vi "Append Paragraph.vi"(0 "PDF Report":T24(xcontrol), 2 "Text":string, 3 "Paragraph indentation":T3, 7 "Image to Add [ ]":T1 {"Scale" format="%#_g %"}, 11 "error in (no error)":errorcluster, 12 "Font":T4={"Name"="", "Size"=-1.0, "Color"=0, "Style"={"Bold"=FALSE, "Italic"=FALSE, "Underline"=FALSE, "Strikeout"=FALSE}}, 14 "Paragraph properties":T8) -> (4 "PDF Report duplicate":T24(xcontrol), 15 "error out":errorcluster)   [LabVIEW 2012]
doc: "Appends text with a <B>line feed</B>, at the end, to the PDF report. This text can be <B>aligned</B> (CENTER, JUSTIFY, LEFT, RIGHT) and <B>indented</B>. \n\nIf <B>Font</B> and <B>Pararaph properties</B> are not specified then the <B>Default font</B> and <B>Default paragraph</B> will be use.\n\nThe data type you wire to the <B>Text</B> input determines the polymorphic instance to use.\n\n<B>FRANÇAIS</B>\nAjoute au rapport PDF du texte sous la forme d'un paragraphe terminé avec un \"<B>Line Feed</B>\". Ce texte peut être <B>aligné</B> (CENTER, JUSTIFY, LEFT, RIGHT) et avoir un <B>renfoncement</B> (gauche et droit) pour tout le paragraphe.\n\nSi la police de caractères <B>Font</B> et les propriétés <B>Pararaph properties</B> ne sont pas spécifiés alors la police par défaut <B>Default font</B> et <B>Default paragraph</B> seront utilisées.\n\nLe type de données que vous connectez au terminal <B>Text</B> détermine l'instance polymorphique utilisée.\n\nDeveloped by Jean-Marc Simard\nCopyright © 2010, Exaprom Inc.\nAll rights reserved.\nLicense: BSD\n\nWith iTextSharp 4.1.6 (http://itextsharp.sourceforge.net)\nunder Mozilla Public License Version 1.1\n(http://www.mozilla.org/MPL/MPL-1.1.html)"
uses:
  Controls/Font cluster.ctl
  Controls/Font size.ctl
  Controls/Font color.ctl
  Controls/Paragraphe cluster.ctl
  Controls/Texte alignement.ctl
  Controls/Line spacing.ctl
  Controls/PDF Report Xcontrol/PDF Report.xctl
  Controls/Paragraph indentation.ctl
  Controls/Image to Add [ ].ctl
  Controls/Image Scale.ctl
  Controls/Phrase or paragraph.ctl
  C:/Users/MaxCorp/Documents/TopPerm - Base/DLL/itextsharp.dll
  DLL/itextsharp.dll
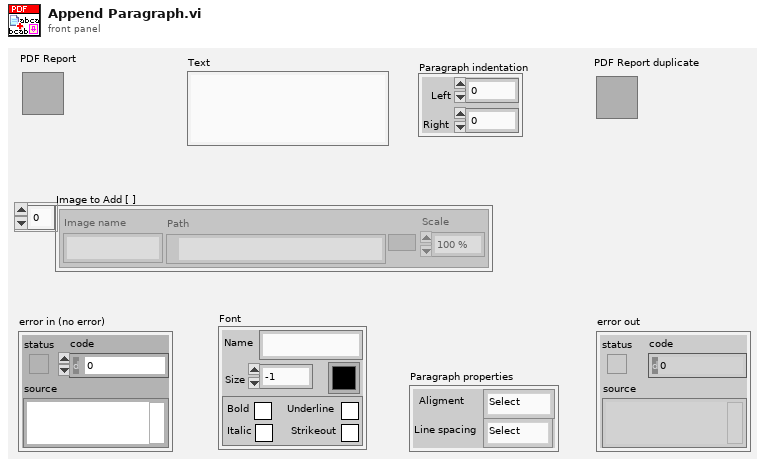
[diagram p1: front panel]
types:
  T1 = typedef "Image to Add [ ].ctl" = cluster{"Image name":string, "Path":path, "Scale":T2}[]
  T2 = typedef "Image Scale.ctl" = sgl
  T3 = typedef "Paragraph indentation.ctl" = cluster{"Left":sgl, "Right":sgl}
  T4 = typedef "Font cluster.ctl" = cluster{"Name":string, "Size":T5, "Color":T6, "Style":cluster{"Bold":bool, "Italic":bool, "Underline":bool, "Strikeout":bool}}
  T5 = typedef "Font size.ctl" = sgl
  T6 = typedef "Font color.ctl" = u32
  T7 = typedef "Unit.ctl" = enum16{"inch", "mm"}
  T8 = typedef "Paragraphe cluster.ctl" = cluster{" Aligment":T9, "Line spacing":T10}
  T9 = typedef "Texte alignement.ctl" = enum16{"Select", "CENTER", "JUSTIFY", "LEFT", "RIGHT"}
  T10 = typedef "Line spacing.ctl" = enum16{"Select", "1.0", "1.5", "2.0"}
  T11 = typedef "Page dimensions.ctl" = cluster{"Start at page":i32, "Orientation":T12, "widht":sgl, "height":sgl, "Margin left":sgl, "Margin right":sgl, "Margin top":sgl, "Margin bottom":sgl}
  T12 = typedef "Page Orientation.ctl" = enum16{"Portrait", "Landscape"}
  T13 = typedef "Image or Table Caption.ctl" = cluster{"Caption":string, "Separator":string, "Position":enum16{"Above", "Below"}}
  T14 = typedef "Header Footer [ ].ctl" = T15[]
  T15 = typedef "Header Footer cluster.ctl" = cluster{"Start page":i32, "Type":T16, "Alignment":T17, "Vertical Alignement":T18, "Image (%)":sgl, "Page #":T19, "Text":string, "Path":string, "Font":T4, "Font refnum":refnum<k24>, "Line":cluster{"Line":T20, "Thickness (points)":sgl, "Colour":T6}}
  T16 = typedef "Header Footer Type.ctl" = enum16{"Select", "Text", "Text + hyperlink", "Page number", "Image", "Image + hyperlink"}
  T17 = typedef "Header footer horiz alignment.ctl" = enum16{"Left", "Center", "Right"}
  T18 = typedef "Cell Vertical alignment.ctl" = enum16{"TOP", "MIDDLE", "BOTTOM"}
  T19 = typedef "Page number.ctl" = cluster{"Text 1":string, "Text 2":string, "Text 3":string}
  T20 = typedef "Header Footer Line.ctl" = enum16{"No line", "Horizontal line"}
  T21 = typedef "Watermark cluster2.ctl" = cluster{"Show? (F)":bool, "Type":enum16{"Image", "Text"}, "Opacity (%)":sgl, "Rotate(°)":sgl, "Position":cluster{"Position":T22, "X":sgl, "Y":sgl}, "Image path":path, "Scaled(%)":sgl, "Image refnum":refnum<k24>, "Text":string, "Font":cluster{"Name":string, "Size":T5, "Color":T6}, "Font refnum":refnum<k24>, "Alignment":T17, "Automatic":bool}
  T22 = typedef "Watermark Position.ctl" = enum16{"Absolute", "Center (page)", "Center (text section)"}
  T23 = typedef "System Fonts.ctl" = cluster{"Font name [ ]":string[], "Font and file names [ ]":cluster{"Font name":string, "File name":string}[]}
  T24 = cluster{"Document":refnum<k24>, "Writer":refnum<k24>, "Default Font":refnum<k24>, "Default Font cluster":T4, "Path":path, "Unit (default = mm)":T7, "Paragraphe cluster":T8, "Pages dimensions [ ]":T11[], "Captions":cluster{"Image":T13, "Image counter":u16, "Table":T13, "Table counter":u16, "Font":T4}, "Header":T14, "Footer":T14, "Watermark ":T21, "Actual VI name":string, "System Fonts":T23}
  T25 = typedef "Phrase or paragraph.ctl" = enum16{"Add to Phrase", "Add to Paragraph", "Create Phrase", "Create Paragraph"}
  T26 = typedef "Image to Add refnum [ ].ctl" = cluster{"Image name":string, "InstanceImage":refnum<k24>}[]
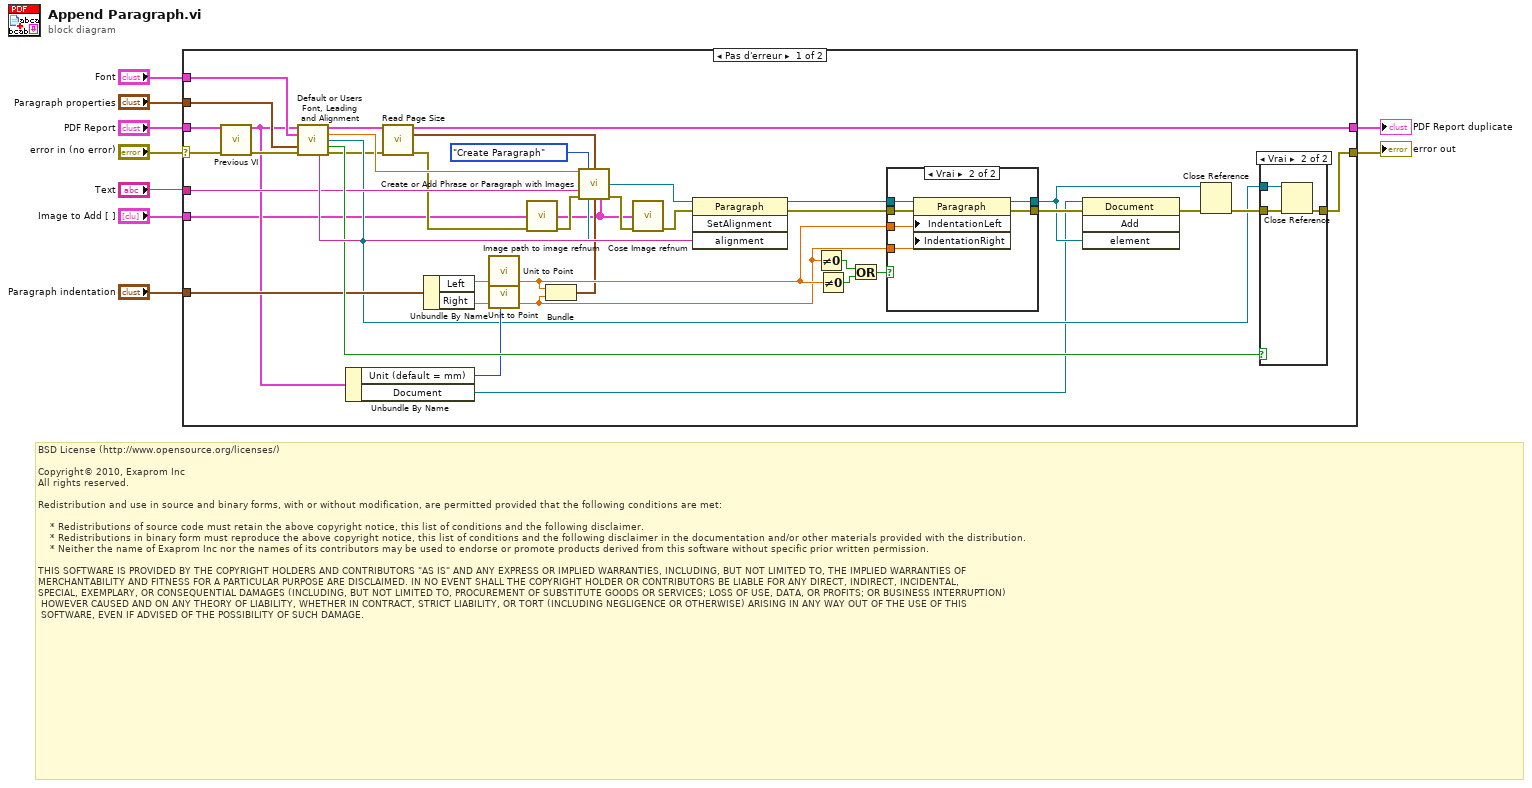
[diagram p0: block diagram]
diagram:
  # "BSD License (http://www.opensource.org/licenses/)\n\nCopyright© 2010, Exaprom Inc\nAll rights reserved.\n\nRedistribution and use in source and binary forms, with or without modification, are permitted provided that the following conditions are met:\n\n    * Redistributions of source code must retain the above copyright notice, this list of conditions and the following disclaimer.\n    * Redistributions in binary form must reproduce the above copyright notice, this list of conditions and the following disclaimer in the documentation and/or other materials provided with the distribution.\n    * Neither the name of Exaprom Inc nor the names of its contributors may be used to endorse or promote products derived from this software without specific prior written permission.\n\nTHIS SOFTWARE IS PROVIDED BY THE COPYRIGHT HOLDERS AND CONTRIBUTORS \"AS IS\" AND ANY EXPRESS OR IMPLIED WARRANTIES, INCLUDING, BUT NOT LIMITED TO, THE IMPLIED WARRANTIES OF \nMERCHANTABILITY AND FITNESS FOR A PARTICULAR PURPOSE ARE DISCLAIMED. IN NO EVENT SHALL THE COPYRIGHT HOLDER OR CONTRIBUTORS BE LIABLE FOR ANY DIRECT, INDIRECT, INCIDENTAL,\nSPECIAL, EXEMPLARY, OR CONSEQUENTIAL DAMAGES (INCLUDING, BUT NOT LIMITED TO, PROCUREMENT OF SUBSTITUTE GOODS OR SERVICES; LOSS OF USE, DATA, OR PROFITS; OR BUSINESS INTERRUPTION)\n HOWEVER CAUSED AND ON ANY THEORY OF LIABILITY, WHETHER IN CONTRACT, STRICT LIABILITY, OR TORT (INCLUDING NEGLIGENCE OR OTHERWISE) ARISING IN ANY WAY OUT OF THE USE OF THIS\n SOFTWARE, EVEN IF ADVISED OF THE POSSIBILITY OF SUCH DAMAGE."
  n1 = case shown="Pas d'erreur" "error in (no error)" {
    selector: "error in (no error)" -> [w21 w64]
    tunnel: "Font" -> [w20 _]
    tunnel: "Text" -> [w31 _]
    tunnel: [w44 w64] -> w8
    tunnel: "PDF Report" -> [w28 w63]
    tunnel: "Paragraph properties" -> [w19 _]
    tunnel: [w10 w63] -> w4
    tunnel: "Paragraph indentation" -> [w39 _]
    tunnel: "Image to Add [ ]" -> [w12 _]
    frame No Error {
      n2 = call "Previous VI.vi"("PDF Report IN"=w28, "error in (no error)"=w21) -> ("PDF Report OUT"=w17:T24, "error out"=w22:errorcluster)  [unwired: 12 out]
      n3 = call "Default or Users Font, Leading and Alignment.vi"("PDF Report"=w17, "Font"=w20, "Paragraphe cluster"=w19, "error in (no error)"=w22) -> ("PDF Report duplicate"=w14:T24, "Leading"=w32:T5, "Font Ref"=w30:refnum<k24>, "Close Font Ref"=w45:bool, "Aligment"=w48:string, "error out"=w16:errorcluster)  [unwired: 6 out]
      n4 = Unbundle By Name(w17) -> ("Unit (default = mm)"=w33:T7, "Document"=w13:refnum<k24>)
      n5 = call "Read Page Size.vi"("PDF Report"=w14, "error in (no error)"=w16) -> ("PDF Report duplicate"=w10:T24, "Text zone (points)"=w18:cluster{"widht":sgl, "height":sgl}, "error out"=w15:errorcluster)  [unwired: 11 out]
      n6 = Unbundle By Name(w39) -> ("Left"=w35:sgl, "Right"=w34:sgl)
      n7 = call "Unit to Point.vi"("X unit"=w35, "Unit (default = mm)"=w33) -> ("X point"=w27:sgl)  [unwired: 7 out]
      n8 = call "Unit to Point.vi"("X unit"=w34, "Unit (default = mm)"=w33) -> ("X point"=w26:sgl)  [unwired: 7 out]
      n9 = call "Image path to image refnum.vi"("Image to Add [ ]"=w12, "error in (no error)"=w15) -> ("Image to Add refnum [ ]"=w11:T26, "error out"=w50:errorcluster)  [unwired: 2 in, 10 out]
      n10 = Bundle("X point"=w27, "X point"=w26) -> (w25:cluster{" X point":sgl, " X point":sgl})  [unwired: 1 out]
      n11 = call "Create or Add Phrase or Paragraph with Images.vi"("Leading"=w32, "Phrase or paragraph"=Phrase_or_paragraph."Create Paragraph", "Text zone (points)"=w18, "Text"=w31, "error in (no error)"=w50, "Font refnum"=w30, "Paragraph indentation (points)"=w25, "Image to Add refnum [ ]"=w11) -> ("Paragraph refnum OUT"=w29:refnum<k24>, "error out"=w24:errorcluster)  [unwired: 3 in, 3 out]
      n12 = call "Cose Image refnum.vi"("Image to Add refnum [ ]"=w11, "error in (no error)"=w24) -> ("error out"=w23:errorcluster)  [unwired: 13 out]
      n13 = invoke class="Paragraph" method="SetAlignment"(reference=w29, error in=w23, "alignment"=w48) -> (reference out=w43:refnum<k24>, error out=w42:errorcluster)  [unwired: 1 in, 2 out]
      n14 = Not Equal To 0?(x=w26) -> (x != 0?=w37:bool)
      n15 = Not Equal To 0?(x=w27) -> (x != 0?=w36:bool)
      n16 = Or(x=w37, y=w36) -> (x .or. y?=w38:bool)
      n17 = case shown="Vrai" w38 {
        tunnel: w43 -> [w52 w58]
        tunnel: w42 -> [w51 w57]
        tunnel: [w51 w56] -> w41
        tunnel: [w52 w55] -> w40
        tunnel: w27 -> [_ w54]
        tunnel: w26 -> [_ w53]
        frame False {
        }
        frame True {
          n18 = property class="Paragraph"(reference=w58, error in=w57, "IndentationLeft"=w54, "IndentationRight"=w53) -> (reference out=w55:refnum<k24>, error out=w56:errorcluster)
        }
      }
      n19 = invoke class="Document" method="Add"(reference=w13, error in=w41, "element"=w40) -> (error out=w47:errorcluster)  [unwired: 1 in, 3 out]
      n20 = Close Reference(reference=w40, error in (no error)=w47) -> (error out=w46:errorcluster)
      n21 = case shown="Vrai" w45 {
        tunnel: [w59 w62] -> w44
        tunnel: w46 -> [w59 w61]
        tunnel: w30 -> [_ w60]
        frame False {
        }
        frame True {
          n22 = Close Reference(reference=w60, error in (no error)=w61) -> (error out=w62:errorcluster)
        }
      }
    }
    frame Error {
    }
  }
  "error out" <- w8
  "PDF Report duplicate" <- w4
